vi "Topas4PublicAPIExample.vi"() -> ()   [LabVIEW 2017]
uses:
  D:/upwork/Laser Measurement Tool/Topas4PublicAPI/NET_SDK/Topas4Lib.dll
  Topas4PublicAPI/NET_SDK/Topas4Lib.dll
panel:
  out "Available interactions":string
  in  "Enter serial number of your own device here":string="Orpheus-HP-Demo-8047"
  # "If you are seeing lots of erros upon downloading and opening this example, this is LabVIEW configuration problem/pseudo-feature.\nCause and solution is described here http://digital.ni.com/public.nsf/allkb/4742EB60B64BE22186257BCE0053B8FD"
  # "You will notice a lot of \"Property node\" vis have \"Ignore Errors inside node\" set to true.\nIt's so because LabView likes to throw strange errors like \"Error 4: end of file\" for reasons that are unknown to me.\nLikely you'll have to do the same."
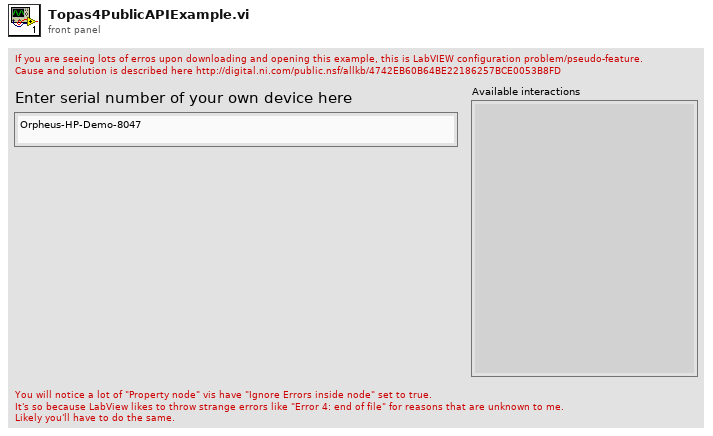
[diagram p1: front panel]
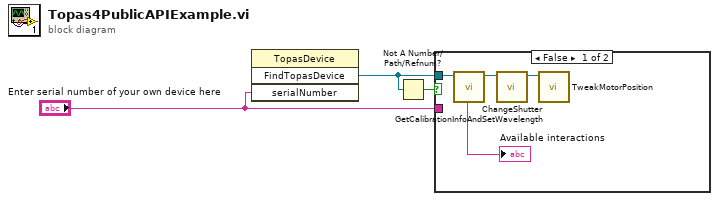
[diagram p0: block diagram]
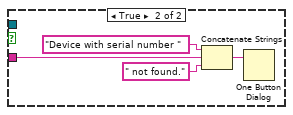
[diagram p2: hidden frame]
diagram:
  n1 = invoke class="TopasDevice" method="FindTopasDevice"("serialNumber"="Enter serial number of your own device here") -> ("FindTopasDevice"=w2:refnum<k24>)  [unwired: 3 in, 3 out]
  n2 = Not A Number/Path/Refnum?(number/path/refnum=w2) -> (NaN/Path/Refnum?=w1:bool)
  n3 = case shown="False" w1 {
    tunnel: w2 -> [w5 _]
    tunnel: "Enter serial number of your own device here" -> [_ w10]
    frame False {
      n4 = call "GetCalibrationInfoAndSetWavelength.vi"("Topas In"=w5) -> ("Topas Out"=w4:refnum<k24>, "Available interactions"=→"Available interactions":string)  [unwired: 7 in, 2 out]
      n5 = call "ChangeShutter.vi"("Topas"=w4) -> ("Topas Out"=w6:refnum<k24>)  [unwired: 10 in]
      n6 = call "TweakMotorPosition.vi"("Topas"=w6) -> ()  [unwired: 10 in, 1 out]
    }
    frame True {
      n7 = Concatenate Strings("Device with serial number " ("string"), w10, " not found.") -> (w8:string)
      n8 = One Button Dialog(message=w8) -> ()  [unwired: 1 in, 1 out]
    }
  }
